vi "FormatTreeStyle.vi"(7 "Format Command":T1, 8 "Error In":errorcluster, 9 "Row Index":i32, 11 "Tree Refnum":refnum<vi>) -> (0 "Error Out":errorcluster)   [LabVIEW 2012]
doc: "SciScan 1.2 160622\nThis VI implements the formatting of table data which includes highlighting, unhighlighting, and modifying visible rows (due to scrolling).\n\n<b>INPUTS</b>\n--------\n<b>Format Command </b> - Formatting action needs to be be taken\n<b>Table references array </b>- Array containing references of the tables of interest\n<b>Row </b>- Row number that needs to be fromatted"
uses:
  CommonResource VIs/FormatTree&TableStyle_Commands.ctl
  <vilib>/Utility/miscctls.llb/LVNodeAndColumnTypeDef.ctl
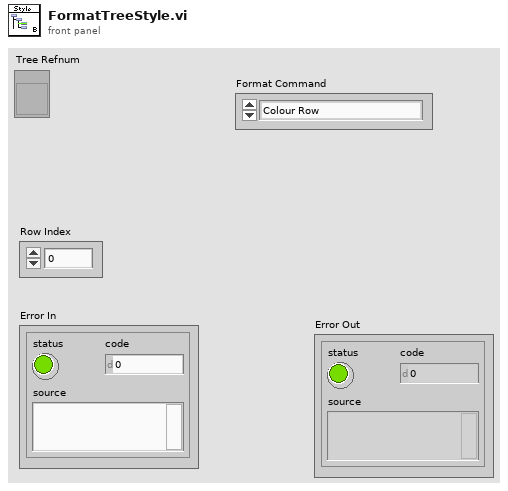
[diagram p1: front panel]
types:
  T1 = typedef "FormatTree&TableStyle_Commands.ctl" = enum16{"Colour Row", "Uncolour Row", "Bold Row", "Unbold Row", "Clear", "UpdateVisibleRows"}
  T2 = typedef "LVNodeAndColumnTypeDef.ctl" = cluster{"Node":string, "Column":i32}
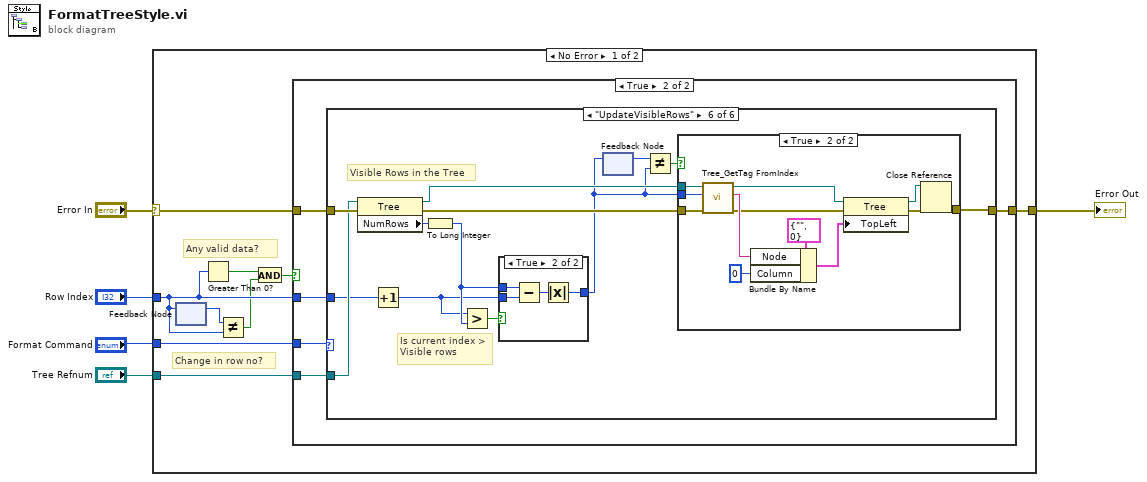
[diagram p0: block diagram]
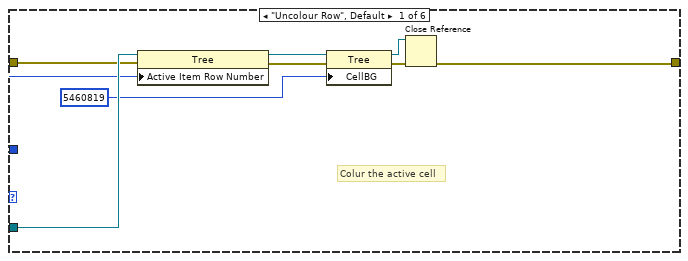
[diagram p3: hidden frame]
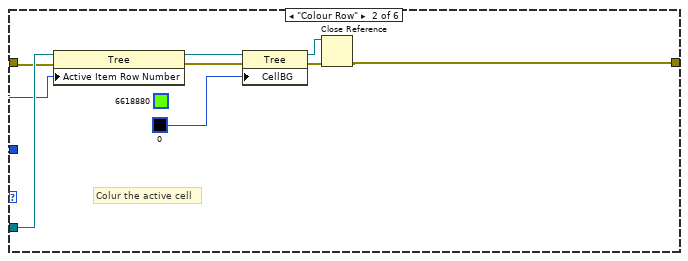
[diagram p4: hidden frame]
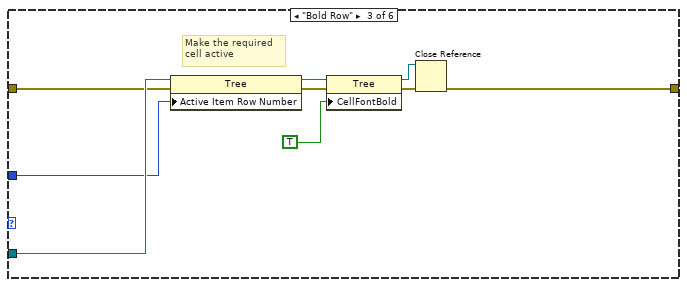
[diagram p5: hidden frame]
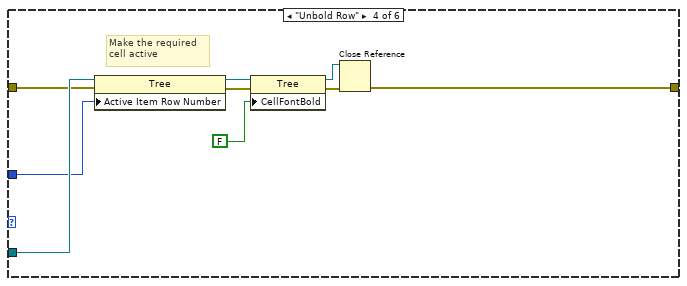
[diagram p6: hidden frame]
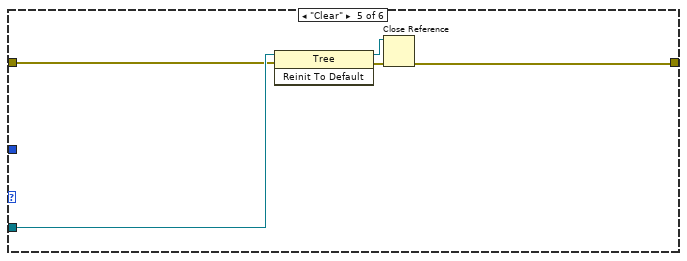
[diagram p7: hidden frame]
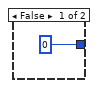
[diagram p9: hidden frame]
diagram:
  n1 = case shown="No Error" "Error In" {
    selector: "Error In" -> [w14 w93]
    tunnel: "Row Index" -> [w9 _]
    tunnel: [w13 w93] -> w3
    tunnel: "Format Command" -> [w12 _]
    tunnel: "Tree Refnum" -> [w11 _]
    frame No Error {
      # "Change in row no?"
      # "Any valid data?"
      n2 = feedback #1() -> (w10:i32)  [unwired: 1 in]
      n3 = feedback-in #1(w9) -> ()
      n4 = Greater Than 0?(x=w9) -> (x > 0?=w7:bool)
      n5 = Not Equal?(x=w10, y=w9) -> (x != y?=w8:bool)
      n6 = And(x=w7, y=w8) -> (x .and. y?=w6:bool)
      n7 = case shown="True" w6 {
        tunnel: w14 -> [w15 w20]
        tunnel: w9 -> [_ w19]
        tunnel: [w15 w18] -> w13
        tunnel: w12 -> [_ w17]
        tunnel: w11 -> [_ w16]
        frame False {
        }
        frame True {
          n8 = case shown="\"UpdateVisibleRows\"" w17 {
            tunnel: w20 -> [w22 w31 w39 w49 w57 w74]
            tunnel: w19 -> [w28 w33 w42 w48 _ w70]
            tunnel: [w23 w32 w41 w51 w58 w68] -> w18
            tunnel: w16 -> [w29 w34 w43 w52 w61 w73]
            frame "Uncolour Row", Default {
              # "Colur the active cell"
              n9 = property class="Tree"(reference=w29, error in=w22, "Active Item Row Number"=w28) -> (reference out=w26:refnum<vi>, error out=w27:errorcluster)
              n10 = property class="Tree"(reference=w26, error in=w27, "CellBG"=u32 5460819 ("Active Cell:Cell Background Color")) -> (reference out=w24:refnum<vi>, error out=w25:errorcluster)
              n11 = Close Reference(reference=w24, error in (no error)=w25) -> (error out=w23:errorcluster)
            }
            frame "Colour Row" {
              (unwired) u32 6618880 ("Background colour")
              # "Colur the active cell"
              n12 = property class="Tree"(reference=w34, error in=w31, "Active Item Row Number"=w33) -> (reference out=w37:refnum<vi>, error out=w38:errorcluster)
              n13 = property class="Tree"(reference=w37, error in=w38, "CellBG"=u32 0 ("Background colour")) -> (reference out=w35:refnum<vi>, error out=w36:errorcluster)
              n14 = Close Reference(reference=w35, error in (no error)=w36) -> (error out=w32:errorcluster)
            }
            frame "Bold Row" {
              # "Make the required cell active"
              n15 = property class="Tree"(reference=w43, error in=w39, "Active Item Row Number"=w42) -> (reference out=w46:refnum<vi>, error out=w47:errorcluster)
              n16 = property class="Tree"(reference=w46, error in=w47, "CellFontBold"=TRUE ("Active Cell:Cell Font:Bold")) -> (reference out=w44:refnum<vi>, error out=w45:errorcluster)
              n17 = Close Reference(reference=w44, error in (no error)=w45) -> (error out=w41:errorcluster)
            }
            frame "Unbold Row" {
              # "Make the required cell active"
              n18 = property class="Tree"(reference=w52, error in=w49, "Active Item Row Number"=w48) -> (reference out=w55:refnum<vi>, error out=w56:errorcluster)
              n19 = property class="Tree"(reference=w55, error in=w56, "CellFontBold"=FALSE ("Active Cell:Cell Font:Bold")) -> (reference out=w53:refnum<vi>, error out=w54:errorcluster)
              n20 = Close Reference(reference=w53, error in (no error)=w54) -> (error out=w51:errorcluster)
            }
            frame "Clear" {
              n21 = invoke class="Tree" method="Reinit To Default"(reference=w61, error in=w57) -> (reference out=w59:refnum<vi>, error out=w60:errorcluster)  [unwired: 1 in, 1 out]
              n22 = Close Reference(reference=w59, error in (no error)=w60) -> (error out=w58:errorcluster)
            }
            frame "UpdateVisibleRows" {
              # "Is current index >\nVisible rows"
              # "Visible Rows in the Tree"
              n23 = property class="Tree"(reference=w73, error in=w74) -> (reference out=w71:refnum<vi>, error out=w72:errorcluster, "NumRows"=w69:u32)
              n24 = Increment(x=w70) -> (x+1=w65:i32)
              n25 = To Long Integer(number=w69) -> (32bit integer=w66:i32)
              n26 = Greater?(x=w65, y=w66) -> (0:w67:bool)
              n27 = case shown="True" w67 {
                tunnel: w66 -> [_ w91]
                tunnel: w65 -> [_ w90]
                tunnel: [0 w89] -> w63
                frame False {
                }
                frame True {
                  n28 = Subtract(x=w91, y=w90) -> (x-y=w92:i32)
                  n29 = Absolute Value(x=w92) -> (abs(x)=w89:i32)
                }
              }
              n30 = feedback #2() -> (w64:i32)  [unwired: 1 in]
              n31 = feedback-in #2(w63) -> ()
              n32 = Not Equal?(x=w64, y=w63) -> (x != y?=w62:bool)
              n33 = case shown="True" w62 {
                tunnel: w72 -> [w75 w87]
                tunnel: w71 -> [_ w86]
                tunnel: [w75 w85] -> w68
                tunnel: w63 -> [_ w76]
                frame False {
                }
                frame True {
                  n34 = call "Tree_GetTag FromIndex.vi"("Error In"=w87, "Index IN"=w76, "Tree Refnum IN"=w86) -> ("Error Out"=w80:errorcluster, "Tag OUT"=w82:string, "Tree Refnum OUT"=w81:refnum<vi>)  [unwired: 6 in]
                  n35 = Bundle By Name(cluster=T2 {"Node"="", "Column"=0} ("Top Left Visible Cell"), "Node"=w82, "Column"=0) -> (w79:T2)
                  n36 = property class="Tree"(reference=w81, error in=w80, "TopLeft"=w79) -> (reference out=w77:refnum<vi>, error out=w78:errorcluster)
                  n37 = Close Reference(reference=w77, error in (no error)=w78) -> (error out=w85:errorcluster)
                }
              }
            }
          }
        }
      }
    }
    frame Error {
    }
  }
  "Error Out" <- w3
